vi "RTS format data file.vi"(0 "Config":T1={"DAQ Settings"={"Trigger Type"=enum."Manual", "Trigger Samples"=0, "Pretrigger Samples"=0, "Trigger Interval"=0.0, "Time Units"=FALSE, "Auto Save"=FALSE, "Sample Rate"=7.0, "Select Analog"=FALSE, "Trigger Value"=0.0, "Trigger Stop Method"=enum."Use Samples Value to Stop Trigger", "Rate Sec/Min"=FALSE, "Save Mode"=enum."Single File", "File Size Limit"=0.0, "Log File Type"=enum."Basic", "Trigger Data Index"=0, "Log Rate"=7.0, "Rate Sec/Min (Log)"=FALSE, "Sample Rate (S/s)"=0.0, "Log Rate (S/s)"=0.0}, "Channels"=[], "Header"={"CA Number"="", "Test Name"="", "Serial Number"="", "Technician"=""}, "Graph Settings"={"Graph Labels"=[], [], [], [], [], [], [], [], [], [], [], [], [], "Graph Toggles"=[], "Axis Toggles"=[], "Graph Range"=enum."1"}, "Test Limits"=[], "All Type Info"=[], "Save Mode"=enum."Single File", "Data Base Path"=path ""} {"DAQ Settings"."Trigger Interval" min=0.0; "DAQ Settings"."Pretrigger Samples" min=0; "DAQ Settings"."Trigger Samples" min=0}, 5 "Start Time":timestamp, 7 "DAQ Rack Name/Version":string) -> (4 "String":string)   [LabVIEW 2019]
uses:
  Type Defs and Controls/Sensor Config.ctl
  Type Defs and Controls/DAQ Settings.ctl
  Type Defs and Controls/Trigger Stop Method.ctl
  Type Defs and Controls/Log File Type.ctl
  Type Defs and Controls/Channel Config.ctl
  Type Defs and Controls/Header.ctl
  Type Defs and Controls/Graph Settings Type Def.ctl
  Type Defs and Controls/Test Limits.ctl
  Type Defs and Controls/All Part Info.ctl
  Type Defs and Controls/Part Info.ctl
panel:
  # "EGU"
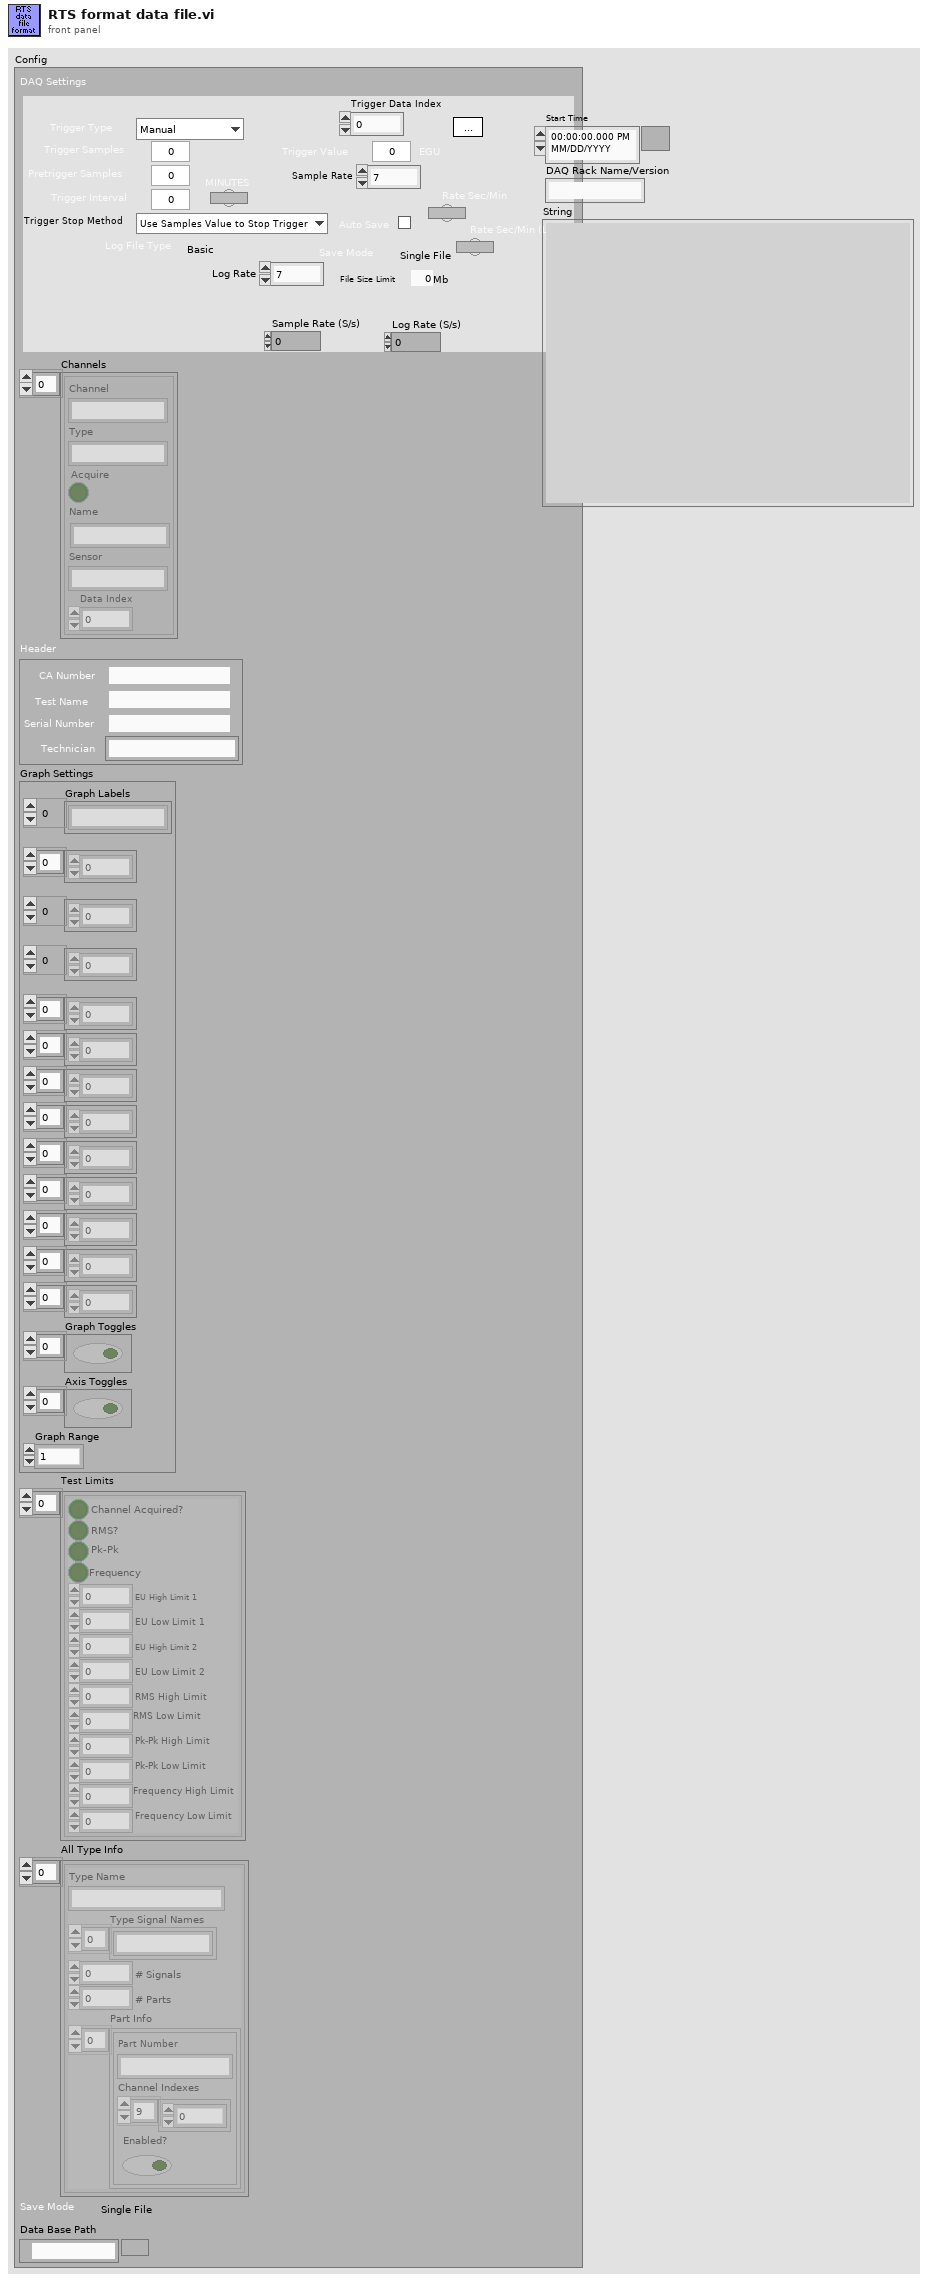
[diagram p1: front panel]
types:
  T1 = typedef "Sensor Config.ctl" = cluster{"DAQ Settings":T2, "Channels":T5[], "Header":T6, "Graph Settings":T7, "Test Limits":T8[], "All Type Info":T9, "Save Mode":enum16{"Single File", "Segmented Files", "New File at Midnight"}, "Data Base Path":path}
  T2 = typedef "DAQ Settings.ctl" = cluster{"Trigger Type":enum16{"Manual", "Timed", "Analog Rising", "Analog Falling"}, "Trigger Samples":i32, "Pretrigger Samples":i32, "Trigger Interval":dbl, "Time Units":bool, "Auto Save":bool, "Sample Rate":dbl, "Select Analog":bool, "Trigger Value":dbl, "Trigger Stop Method":T3, "Rate Sec/Min":bool, "Save Mode":enum16{"Single File", "Segmented Files", "New File at Midnight"}, "File Size Limit":dbl, "Log File Type":T4, "Trigger Data Index":u32, "Log Rate":dbl, "Rate Sec/Min (Log)":bool, "Sample Rate (S/s)":dbl, "Log Rate (S/s)":dbl}
  T3 = typedef "Trigger Stop Method.ctl" = enum16{"Use Samples Value to Stop Trigger", "Use Threshold to Stop Trigger"}
  T4 = typedef "Log File Type.ctl" = enum16{"Basic", "RTS"}
  T5 = typedef "Channel Config.ctl" = cluster{"Channel":string, "Type":string, "Acquire":bool, "Name":string, "Sensor":string, "Data Index":u32}
  T6 = typedef "Header.ctl" = cluster{"CA Number":string, "Test Name":string, "Serial Number":string, "Technician":string}
  T7 = typedef "Graph Settings Type Def.ctl" = cluster{"Graph Labels":string[], u8[], i16[], u32[], u8[], u8[], u8[], u32[], u8[], u8[], u8[], dbl[], dbl[], "Graph Toggles":bool[], "Axis Toggles":bool[], "Graph Range":enum16{"1", "2", "3", "4", "5", "10", "15", "30", "60"}}
  T8 = typedef "Test Limits.ctl" = cluster{"Channel Acquired?":bool, "RMS?":bool, "Pk-Pk":bool, "Frequency":bool, "EU High Limit 1":dbl, "EU Low Limit 1":dbl, "EU High Limit 2":dbl, "EU Low Limit 2":dbl, "RMS High Limit":dbl, "RMS Low Limit":dbl, "Pk-Pk High Limit ":dbl, "Pk-Pk Low Limit":dbl, "Frequency High Limit":dbl, "Frequency Low Limit":dbl}
  T9 = typedef "All Part Info.ctl" = cluster{"Type Name":string, "Type Signal Names":string[], "# Signals":i32, "# Parts":i32, "Part Info":T10[]}[]
  T10 = typedef "Part Info.ctl" = cluster{"Part Number":string, "Channel Indexes":u16[], "Enabled?":bool}
  T11 = cluster{"Type Name":string, "Type Signal Names":string[], "# Signals":i32, "# Parts":i32, "Part Info":T10[]}
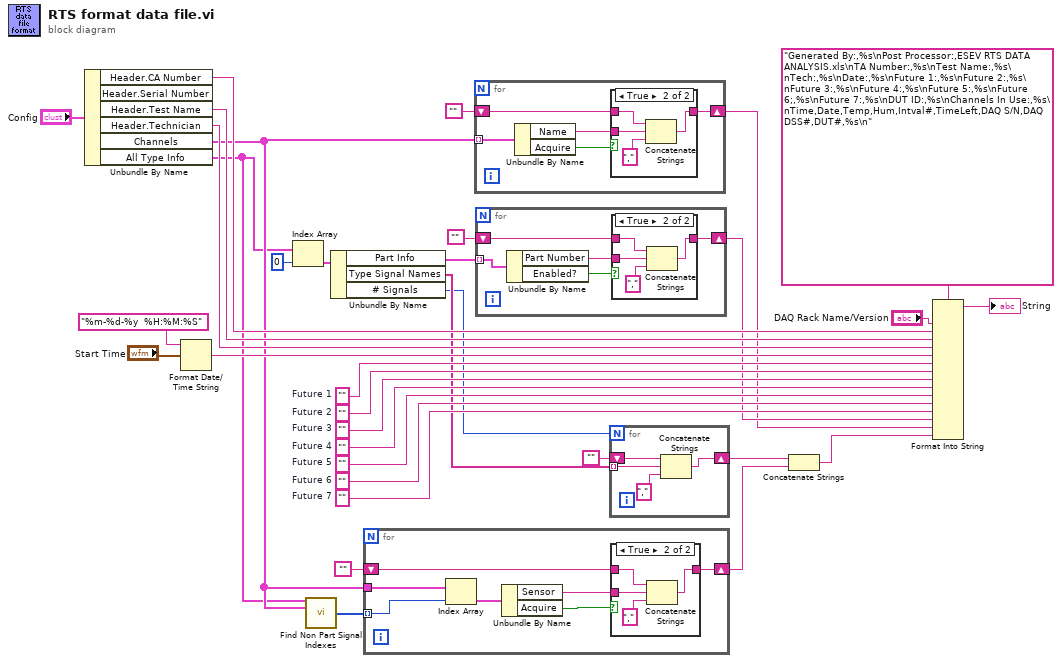
[diagram p0: block diagram]
diagram:
  w20 = ""  # Future 7
  w21 = ""  # Future 6
  w22 = ""  # Future 5
  w23 = ""  # Future 4
  w24 = ""  # Future 3
  w25 = ""  # Future 2
  w26 = ""  # Future 1
  n1 = Unbundle By Name("Config") -> ("Header.CA Number"=w31:string, "Header.Test Name"=w30:string, "Header.Technician"=w12:string, "Channels"=w5:T5[], "All Type Info"=w2:T9)  [unwired: 1 out]
  n2 = Format Date/Time String(time format string (%c)="%m-%d-%y  %H:%M:%S", seconds (now)="Start Time") -> (date/time string=w27:string)  [unwired: 1 in]
  n3 = Index Array(array=w2, index=0) -> (element=w18:T11)
  n4 = call "Find Non Part Signal Indexes.vi"("All Type Info"=w2, "Channels"=w5) -> ("Non Part Indexes (description)"=w1:i32[])  [unwired: 11 in, 2 out]
  n5 = Unbundle By Name(w18) -> ("Part Info"=w14:T10[], "Type Signal Names"=w9:string[], "# Signals"=w6:i32)
  n6 = for {
    tunnel: w5 -> [w40]
    shift-right: [w38] -> w4
    shift-left: "" -> [w37]
    tunnel: w1 -> [w35] mode=indexing
    n7 = Index Array(array=w40, index=w35) -> (element=w39:T5)
    n8 = Unbundle By Name(w39) -> ("Sensor"=w41:string, "Acquire"=w36:bool)
    n9 = case shown="True" w36 {
      tunnel: w41 -> [_ w44]
      tunnel: [w42 w46] -> w38
      tunnel: w37 -> [w42 w45]
      frame False {
      }
      frame True {
        n10 = Concatenate Strings(w45, w44, "," ("string")) -> (w46:string)
      }
    }
  }
  n11 = for {
    tunnel: w5 -> [w51] mode=indexing
    shift-right: [w48] -> w10
    shift-left: "" -> [w49]
    n12 = Unbundle By Name(w51) -> ("Name"=w50:string, "Acquire"=w47:bool)
    n13 = case shown="True" w47 {
      tunnel: w50 -> [_ w56]
      tunnel: w49 -> [w52 w55]
      tunnel: [w52 w53] -> w48
      frame False {
      }
      frame True {
        n14 = Concatenate Strings(w55, w56, "," ("string")) -> (w53:string)
      }
    }
  }
  n15 = for {
    tunnel: w14 -> [w61] mode=indexing
    shift-right: [w58] -> w11
    shift-left: "" -> [w59]
    n16 = Unbundle By Name(w61) -> ("Part Number"=w60:string, "Enabled?"=w57:bool)
    n17 = case shown="True" w57 {
      tunnel: w60 -> [_ w66]
      tunnel: w59 -> [w62 w65]
      tunnel: [w62 w63] -> w58
      frame False {
      }
      frame True {
        n18 = Concatenate Strings(w65, w66, "," ("string")) -> (w63:string)
      }
    }
  }
  n19 = for {
    N: w6 -> [_]
    tunnel: w9 -> [w68] mode=indexing
    shift-right: [w70] -> w8
    shift-left: "" -> [w69]
    n20 = Concatenate Strings(w69, w68, "," ("string")) -> (w70:string)
  }
  n21 = Concatenate Strings(w8, w4) -> (w7:string)
  n22 = Format Into String(format string="Generated By:,%s\nPost Processor:,ESEV RTS DATA ANALYSIS.xls\nTA Number:,%s\nTest Name:,%s\nTech:,%s\nDate:,%s\nFuture 1:,%s\nFuture 2:,%s\nFuture 3:,%s\nFuture 4:,%s\nFuture 5:,%s\nFuture 6;,%s\nFuture 7:,%s\nDUT ID:,%s\nChannels In Use:,%s\nTime,Date,Temp,Hum,Intval#,TimeLeft,DAQ S/N,DAQ DSS#,DUT#,%s\n", "DAQ Rack Name/Version", w31, w30, w12, w27, w26, w25, w24, w23, w22, w21, w20, w11, w10, w7) -> (resulting string=→"String":string)  [unwired: 2 in, 1 out]
